vi "calculate_item_names_width.vi"(8 "error in (no error)":errorcluster, 11 "listbox_reference":refnum<vi>) -> (0 "error out":errorcluster, 4 "width []":u32[](array[numeric]), 6 "height []":u32[](array[numeric]))   [LabVIEW 2015, in "lv-pagination.lvlib"]
uses:
  lv-pagination.lvlib
  <vilib>/Utility/miscctls.llb/LVRowAndColumnTypeDef.ctl
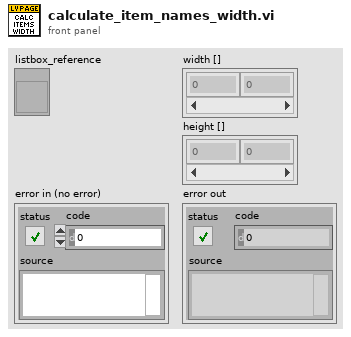
[diagram p1: front panel]
types:
  T1 = enum16{"User-specified Font", "Application Font", "System Font", "Dialog Font"}
  T2 = typedef "LVRowAndColumnTypeDef.ctl" = cluster{"Row":i32, "Column":i32}
  T3 = cluster{"CellFontName":string, "CellFontSize":u32, "CellFontStrike":bool, "CellFontItalic":bool, "CellFontUnder":bool, bool, bool, "CellFontBold":bool}
  T4 = cluster{"left":i16, "top":i16, "right":i16, "bottom":i16}
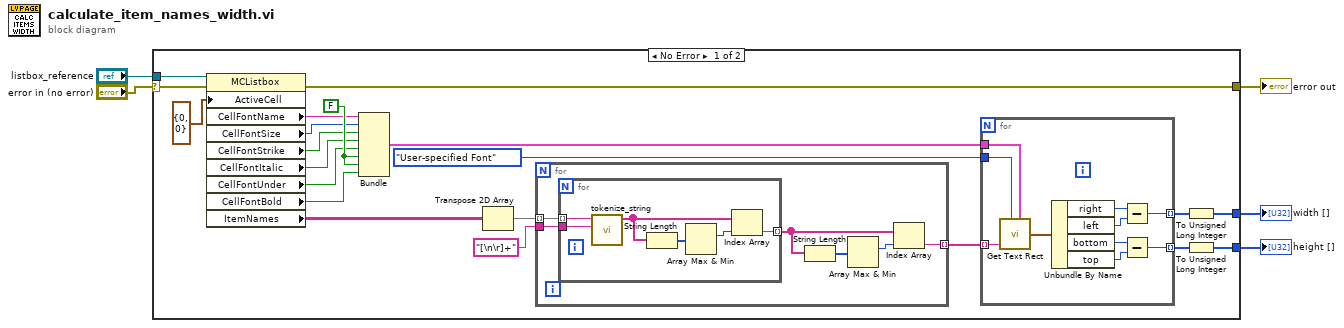
[diagram p0: block diagram]
diagram:
  n1 = case shown="No Error" "error in (no error)" {
    selector: "error in (no error)" -> [w25 w49]
    tunnel: "listbox_reference" -> [w26 _]
    tunnel: [w24 w49] -> w3
    tunnel: [w7 _] -> w2
    tunnel: [w6 _] -> w1
    frame No Error {
      w21 = FALSE
      n2 = property on="Property Node" class="MCListbox"(reference=w26, error in=w25, "ActiveCell"=T2 {"Row"=0, "Column"=0} ("Active Cell:Active Cell")) -> (error out=w24:errorcluster, "CellFontName"=w15:string, "CellFontSize"=w16:u32, "CellFontStrike"=w17:bool, "CellFontItalic"=w18:bool, "CellFontUnder"=w19:bool, "CellFontBold"=w20:bool, "ItemNames"=w13:string[][])  [unwired: 1 out]
      n3 = Bundle("CellFontName"=w15, "CellFontSize"=w16, "CellFontStrike"=w17, "CellFontItalic"=w18, "CellFontUnder"=w19, w21, w21, "CellFontBold"=w20) -> (w12:T3)  [unwired: 1 in]
      n4 = Transpose 2D Array(2D array=w13) -> (transposed array=w23:string[][])
      n5 = for {
        tunnel: "[\n\r]+" ("delimiter ([\\s\\t\\n\\r]+)") -> [w42]
        tunnel: w23 -> [w41] mode=indexing
        tunnel: [w37] -> w10 mode=indexing
        n6 = for {
          tunnel: w41 -> [w44] mode=indexing
          tunnel: [w46] -> w38 mode=indexing
          tunnel: w42 -> [w43]
          n7 = call "tokenize_string.vi"("delimiter"=w43, "input_string"=w44) -> ("delimited_string []"=w45:string[])  [unwired: 8 in, 1 out]
          n8 = String Length(string=w45) -> (length=w47:i32[])
          n9 = Array Max & Min(array=w47) -> (max index (indices)=w48:i32)  [unwired: 3 out]
          n10 = Index Array(array=w45, index=w48) -> (element=w46:string)
        }
        n11 = String Length(string=w38) -> (length=w40:i32[])
        n12 = Array Max & Min(array=w40) -> (max index (indices)=w39:i32)  [unwired: 3 out]
        n13 = Index Array(array=w38, index=w39) -> (element=w37:string)
      }
      n14 = for {
        tunnel: w10 -> [w33] mode=indexing
        tunnel: w12 -> [w32]
        tunnel: [w31] -> w9 mode=indexing
        tunnel: T1."User-specified Font" ("desired font(Application)") -> [w30]
        tunnel: [w27] -> w8 mode=indexing
        n15 = call <vilib>:"Get Text Rect.vi"("desired font(Application)"=w30, "text"=w33, "[user-specified font]"=w32) -> ("rect"=w36:T4)  [unwired: 6 in]
        n16 = Unbundle By Name(w36) -> ("right"=w35:i16, "left"=w34:i16, "bottom"=w29:i16, "top"=w28:i16)
        n17 = Subtract(x=w35, y=w34) -> (x-y=w31:i16)
        n18 = Subtract(x=w29, y=w28) -> (x-y=w27:i16)
      }
      n19 = To Unsigned Long Integer(number=w9) -> (unsigned 32bit integer=w7:u32[])
      n20 = To Unsigned Long Integer(number=w8) -> (unsigned 32bit integer=w6:u32[])
    }
    frame Error {
    }
  }
  "error out" <- w3
  "width []" <- w2
  "height []" <- w1
